vi "Update msg.vi"(8 "error in (no error)":errorcluster, 10 "Update Mensaje":string, 11 "Mensaje Actor in":refnum<class "Mensaje Actor.lvclass">) -> (0 "error out":errorcluster, 3 "Mensaje Actor out":refnum<class "Mensaje Actor.lvclass">)   [LabVIEW 2019, in "Mensaje Actor.lvlib" / "Mensaje Actor.lvclass"]
uses:
  Mensaje Actor.lvclass
  Mensaje Actor.lvclass/Mensaje Actor.ctl
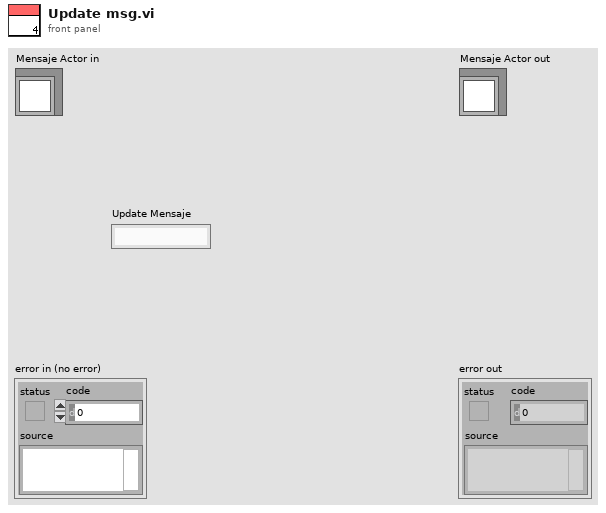
[diagram p1: front panel]
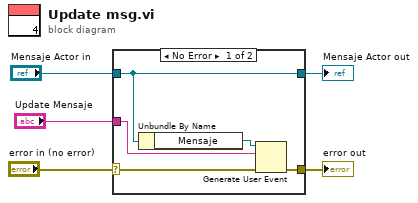
[diagram p0: block diagram]
diagram:
  n1 = case shown="No Error" "error in (no error)" {
    selector: "error in (no error)" -> [w8 w12]
    tunnel: [w7 w12] -> w4
    tunnel: [w10 w11] -> w2
    tunnel: "Mensaje Actor in" -> [w10 w11]
    tunnel: "Update Mensaje" -> [w6 _]
    frame No Error {
      n2 = Unbundle By Name(w10) -> ("Mensaje"=w9:refnum<user-event>)
      n3 = Generate User Event(user event=w9, event data cluster=w6, error in=w8) -> (error out=w7:errorcluster)  [unwired: 1 in, 1 out]
    }
    frame Error {
    }
  }
  "error out" <- w4
  "Mensaje Actor out" <- w2
